vi "Configure Function Delay.vi"(7 "Delay Time (0 s)":dbl, 8 "error in (no error)":errorcluster, 9 "Operand Name (0: Channel 1)":i32(ring) items=["Channel 1", "Channel 2", "Channel 3", "Channel 4", "Differential 1", "Differential 2", "Common 1", "Common 2", "Function 1", "Function 2", "Function 3", "Function 4", "Function 5", "Function 6", "Function 7", "Function 8", "Function 9", "Function 10", "Function 11", "Function 12", "Function 13", "Function 14", "Function 15", "Function 16", "Memory 1", "Memory 2", "Memory 3", "Memory 4", "MTRend", "MSPectrum"], 10 "Function Channel (1: Function 1)":i32(ring)=1 items=["Function 1"=1, "Function 2"=2, "Function 3"=3, "Function 4"=4, "Function 5"=5, "Function 6"=6, "Function 7"=7, "Function 8"=8, "Function 9"=9, "Function 10"=10, "Function 11"=11, "Function 12"=12, "Function 13"=13, "Function 14"=14, "Function 15"=15, "Function 16"=16], 11 "VISA resource name":refnum<visa-resource-name>) -> (0 "error out":errorcluster, 3 "VISA resource name out":refnum<visa-resource-name>)   [LabVIEW 2020, in "Agilent 90000 Series.lvlib"]
doc: "Adds the provided time to the X origin of the source waveform, effectively shifting the function waveform in time.\n\n<b>Note:</b>\nThis VI is new in firmware version 4.30."
uses:
  Agilent 90000 Series.lvlib
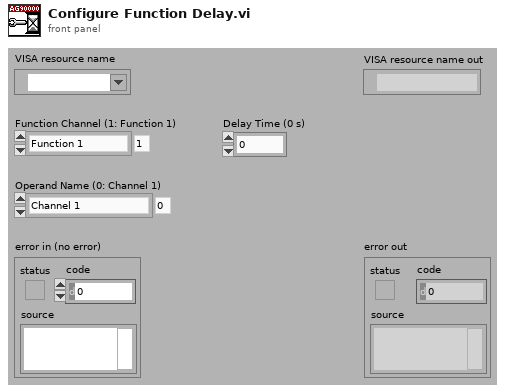
[diagram p1: front panel]
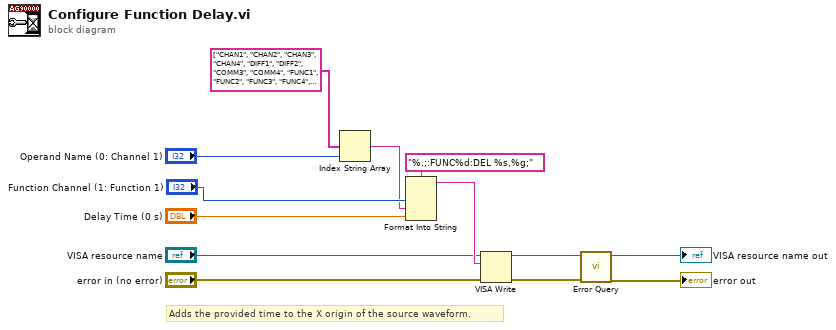
[diagram p0: block diagram]
diagram:
  # "Adds the provided time to the X origin of the source waveform."
  n1 = Index String Array(1:"Operand Name (0: Channel 1)", 2:string[] ["CHAN1", "CHAN2", "CHAN3", "CHAN4", "DIFF1", "DIFF2", "COMM3", "COMM4", "FUNC1", "FUNC2", "FUNC3", "FUNC4", "FUNC5", "FUNC6", "FUNC7", "FUNC8", "FUNC9", "FUNC10", "FUNC11", "FUNC12", "FUNC13", "FUNC14", "FUNC15", "FUNC16", "WMEM1", "WMEM2", "WMEM3", "WMEM4", "MTR", "MSP"] ("string array")) -> (0:w1:string)  [unwired: 1 in]
  n2 = Format Into String(format string="%.;:FUNC%d:DEL %s,%g;", "Function Channel (1: Function 1)", w1, "Delay Time (0 s)") -> (resulting string=w10:string)  [unwired: 2 in, 1 out]
  n3 = VISA Write(VISA resource name="VISA resource name", write buffer=w10, error in (no error)="error in (no error)") -> (VISA resource name out=w7:refnum<visa-resource-name>, error out=w6:errorcluster)  [unwired: 1 out]
  n4 = call "Error Query.vi"("error in (no error)"=w6, "VISA resource name"=w7) -> ("error out"=→"error out":errorcluster, "VISA resource name out"=→"VISA resource name out":refnum<visa-resource-name>)  [unwired: 6 in, 2 out]
